vi "TDT-Select Block.vi"(0 "Data":T2={"TTankX"=refnum, "TDevAccX"=refnum, "LastTime"=0.0, "error"={"status"=FALSE, "code"=0, "source"=""}, "Block Name"="", "Circuit Tag"="", "Tank Name"="", "NumTicks"=0, "LastTick"=0.0, "Idle?"=FALSE, "Wait (ms)"=1000, "LastArtf"=0.0, "LastTosc"=0.0}, 7 "Mode":T1, 11 "error in (no error)":errorcluster, 12 "milliseconds to wait":u32=1000) -> (6 "TankName":string, 8 "Block Name":string, 15 "error out":errorcluster)   [LabVIEW 2015]
uses:
  TDT Interface Data.ctl
  TDT-Sys Mode Enum.ctl
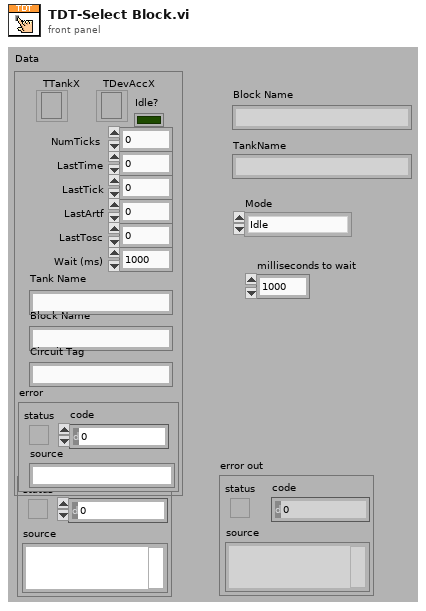
[diagram p1: front panel]
types:
  T1 = typedef "TDT-Sys Mode Enum.ctl" = enum16{"Idle", "Standby", "Preview", "Record"}
  T2 = typedef "TDT Interface Data.ctl" = cluster{"TTankX":refnum<k7>, "TDevAccX":refnum<k7>, "LastTime":dbl, "error":errorcluster, "Block Name":string, "Circuit Tag":string, "Tank Name":string, "NumTicks":i32, "LastTick":dbl, "Idle?":bool, "Wait (ms)":u32, "LastArtf":dbl, "LastTosc":dbl}
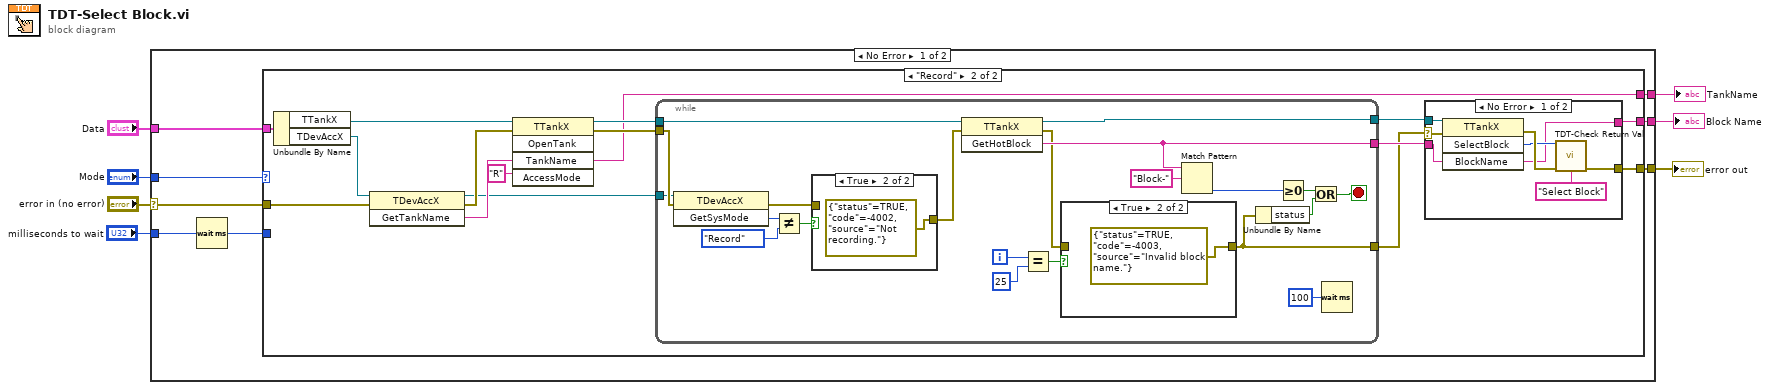
[diagram p0: block diagram]
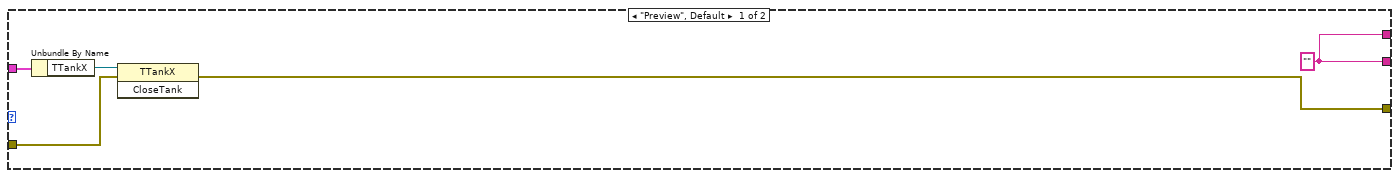
[diagram p2: hidden frame]
diagram:
  n1 = case shown="No Error" "error in (no error)" {
    selector: "error in (no error)" -> [w12 w71]
    tunnel: [w15 w71] -> w6
    tunnel: "Data" -> [w14 _]
    tunnel: [w13 _] -> w4
    tunnel: "Mode" -> [w11 _]
    tunnel: [w10 _] -> w2
    tunnel: "milliseconds to wait" -> [w9 _]
    frame No Error {
      n2 = Wait (ms)(milliseconds to wait=w9) -> (millisecond timer value=w8:u32)
      n3 = case shown="\"Record\"" w11 {
        tunnel: [w17 w36] -> w15
        tunnel: w14 -> [w20 w35]
        tunnel: [w16 w32] -> w13
        tunnel: w12 -> [w18 w30]
        tunnel: [w16 w23] -> w10
        tunnel: w8 -> [_ _]
        frame "Preview", Default {
          w16 = "" ("BlockName")
          n4 = Unbundle By Name(w20) -> ("TTankX"=w19:refnum<k7>)
          n5 = invoke class="TTankX" method="CloseTank"(reference=w19, error in=w18) -> (error out=w17:errorcluster)  [unwired: 1 in, 2 out]
        }
        frame "Record" {
          n6 = Unbundle By Name(w35) -> ("TTankX"=w29:refnum<k7>, "TDevAccX"=w31:refnum<k7>)
          n7 = invoke class="TDevAccX" method="GetTankName"(reference=w31, error in=w30) -> (reference out=w21:refnum<k7>, error out=w26:errorcluster, "GetTankName"=w27:string)  [unwired: 1 in]
          n8 = invoke class="TTankX" method="OpenTank"(reference=w29, error in=w26, "TankName"=w27, "AccessMode"="R") -> (reference out=w28:refnum<k7>, error out=w24:errorcluster, "TankName"=w23:string)  [unwired: 1 in, 2 out]
          n9 = while {
            tunnel: [w66] -> w34
            tunnel: [w63] -> w33
            tunnel: w28 -> [w65]
            tunnel: w24 -> [w52]
            tunnel: [w53] -> w22
            tunnel: w21 -> [w51]
            i -> [w60]
            stop <- w57 stop-if-true
            n10 = invoke class="TDevAccX" method="GetSysMode"(reference=w51, error in=w52) -> (error out=w47:errorcluster, "GetSysMode"=w50:i32)  [unwired: 1 in, 1 out]
            n11 = Not Equal?(x=w50, y=TDT-Sys_Mode_Enum."Record" ("Mode")) -> (x != y?=w48:bool)
            n12 = case shown="True" w48 {
              tunnel: w47 -> [w67 _]
              tunnel: [w67 errorcluster {"status"=TRUE, "code"=-4002, "source"="Not recording."} ("error out")] -> w46
              frame False {
              }
              frame True {
              }
            }
            n13 = invoke class="TTankX" method="GetHotBlock"(reference=w65, error in=w46) -> (reference out=w66:refnum<k7>, error out=w55:errorcluster, "GetHotBlock"=w63:string)  [unwired: 1 in]
            n14 = Equal?(x=w60, y=25) -> (x = y?=w56:bool)
            n15 = case shown="True" w56 {
              tunnel: w55 -> [w69 _]
              tunnel: [w69 errorcluster {"status"=TRUE, "code"=-4003, "source"="Invalid block name."} ("error out")] -> w53
              frame False {
              }
              frame True {
              }
            }
            n16 = Match Pattern(string=w63, regular expression="Block-") -> (offset past match=w61:i32)  [unwired: 1 in, 3 out]
            n17 = Unbundle By Name(w53) -> ("status"=w54:bool)
            n18 = Greater Or Equal To 0?(x=w61) -> (x >= 0?=w58:bool)
            n19 = Or(x=w58, y=w54) -> (x .or. y?=w57:bool)
            n20 = Wait (ms)(milliseconds to wait=u32 100) -> ()  [unwired: 1 out]
          }
          n21 = case shown="No Error" w22 {
            selector: w22 -> [w37 w45]
            tunnel: [w43 w45] -> w36
            tunnel: w34 -> [w42 _]
            tunnel: w33 -> [w41 _]
            tunnel: [w38 _] -> w32
            frame No Error {
              n22 = invoke class="TTankX" method="SelectBlock"(reference=w42, error in=w37, "BlockName"=w41) -> (error out=w40:errorcluster, "SelectBlock"=w39:i32, "BlockName"=w38:string)  [unwired: 1 in, 1 out]
              n23 = call "TDT-Check Return Val.vi"("Return Val"=w39, "error in (no error)"=w40, "source"="Select Block" ("Message")) -> ("error out"=w43:errorcluster)  [unwired: 12 in]
            }
            frame Error {
            }
          }
        }
      }
    }
    frame Error {
    }
  }
  "error out" <- w6
  "Block Name" <- w4
  "TankName" <- w2
